vi "cs-scanning-condition-disable-example.vi"() -> ()   [LabVIEW 2017]
uses:
  raster-scan-params.ctl
  controls/PI-params.ctl
  controls/boolean_info.ctl
  <vilib>/rvi/Emulation/niFpgaGetClockAttributes.vi
  <vilib>/rvi/Emulation/niFpgaSctlEmulationGetInTimedLoop.vi
  <vilib>/rvi/Emulation/niFpgaEmulationReportErrorSimple.vi
  <vilib>/rvi/eio/common/nirviEmuTemplateMethod_errors.vi
  <vilib>/rvi/Emulation/niFpgaProcessEmulError.vi
  <vilib>/rvi/Emulation/niFpgaEmulationIsFPGAContextNoSignature.vi
  <vilib>/rvi/DataTransferAndStorage/Container/Common/niFpgaContainerGetUniqueNameForEmu.vi
  <vilib>/rvi/Memory/Memory_Emulation/niFpgaMemoryEmulationCacheClearOnFirstRun.vi
  <vilib>/rvi/Memory/Memory_Emulation/nirvimemoryEmulationManagerCache_MakeExclusive.vi
  <vilib>/rvi/Memory/Memory_Emulation/niFpgaMemoryEmulationValidateCache.vi
  <vilib>/rvi/Memory/Memory_Emulation/nirvimemoryEmulationManagerCache_InsertValue.vi
  <vilib>/Utility/error.llb/Clear Errors.vi
  <vilib>/rvi/Memory/Memory_Emulation/nirvimemoryEmulationManagerCache_ReleaseExclusive.vi
  <vilib>/rvi/Memory/Memory_Emulation/nirvimemoryEmulationManagerCache_GetValue.vi
  <vilib>/rvi/Memory/Memory_Emulation/nirvimemoryEmulationManagerCache_SetValue.vi
  <vilib>/rvi/Emulation/niFpgaCriticalErrorInLSC.vi
  <vilib>/eio/EIONode/EIONode.xnode
  <vilib>/rvi/DataTransferAndStorage/Container/XNode/niFpgaContainer.xnode
  <vilib>/rvi/DataTransferAndStorage/Register/Emulation/niFpgaRegisterEmulation.vi
  FPGA-data-logging.lvlib
  libimaging-cs.lvlib
panel:
  out "number-settled-samples-Z":i16
  in  "Z-error-threshold":sgl format="%#_13g"
  in  "Z-settled-samples\nthreshold":i16
  in  "Ki-z-absolute":sgl
  in  "z_UP 2":fxp<+/-,16,5>
  in  "z_UP":fxp<+/-,16,5>
  out "Current Case":i16
  out "boolean \nindicators":T1
  out "z-u(k)":sgl
  in  "ABORT":bool
  out "read fifo timeout":bool
  in  "u_z max":sgl
  in  "numEntities":i16
  in  "raster-scan-params":T2={"TsTicks"=1600, "Stop"=TRUE, "TOL"=0.3, "ramp-rate"=0.0, "z-u-max"=5.0, "PI-params"={"Ki"=0.001, "setpoint"=0.0}} {"z-u-max" format="%#_13g"; "TOL" format="%#_13g"}
  out "e(0) (threshhold init)":fxp<+/-,16,5>
  in  "init Z up":fxp<+/-,16,5>
  in  "trigger-0":bool
  in  "zup-N":i16
  out "number-settled-samples-y":i16
  out "number-settled-samples-x":i16
  in  "error-threshold":sgl format="%#_13g"
  in  "settled-samples\nthreshold":i16
  in  "Ki-xy":sgl=0.001 format="%#_13g"
  in  "xy-bound":sgl
  in  "initial case":i16=2
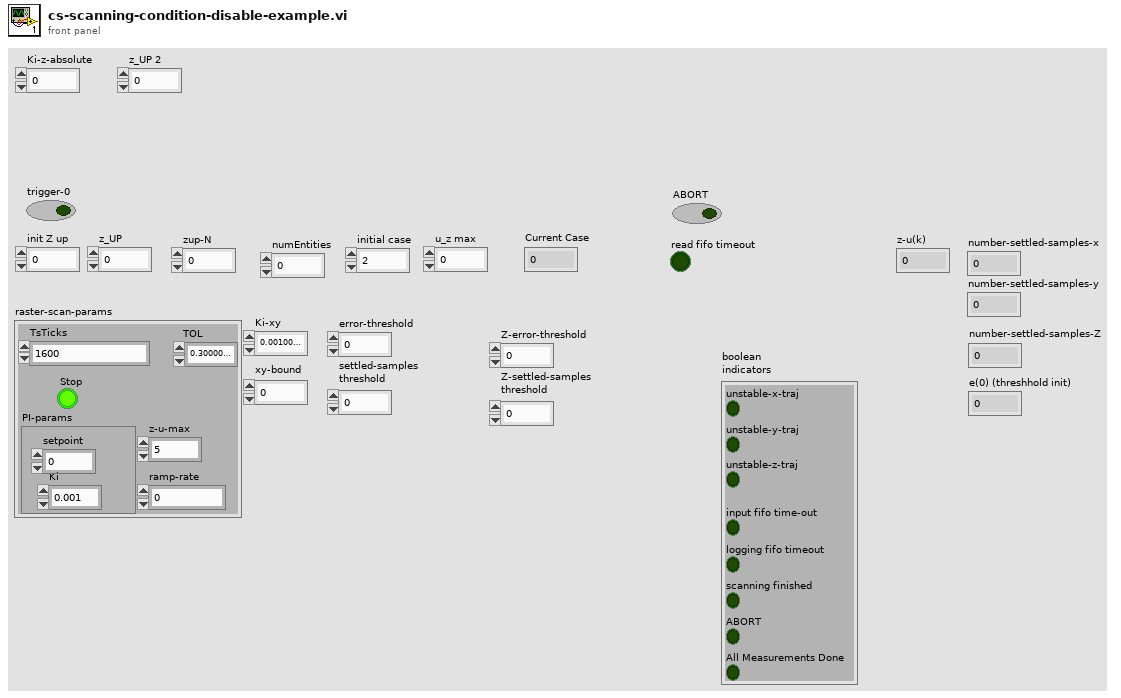
[diagram p1: front panel]
types:
  T1 = typedef "boolean_info.ctl" = cluster{"unstable-z-traj":bool, "input fifo time-out":bool, "logging fifo timeout":bool, "scanning finished":bool, "unstable-x-traj":bool, "unstable-y-traj":bool, "ABORT":bool, "All Measurements Done":bool}
  T2 = typedef "raster-scan-params.ctl" = cluster{"TsTicks":u32, "Stop":bool, "TOL":sgl, "ramp-rate":sgl, "z-u-max":sgl, "PI-params":T3}
  T3 = typedef "PI-params.ctl" = cluster{"Ki":sgl, "setpoint":sgl}
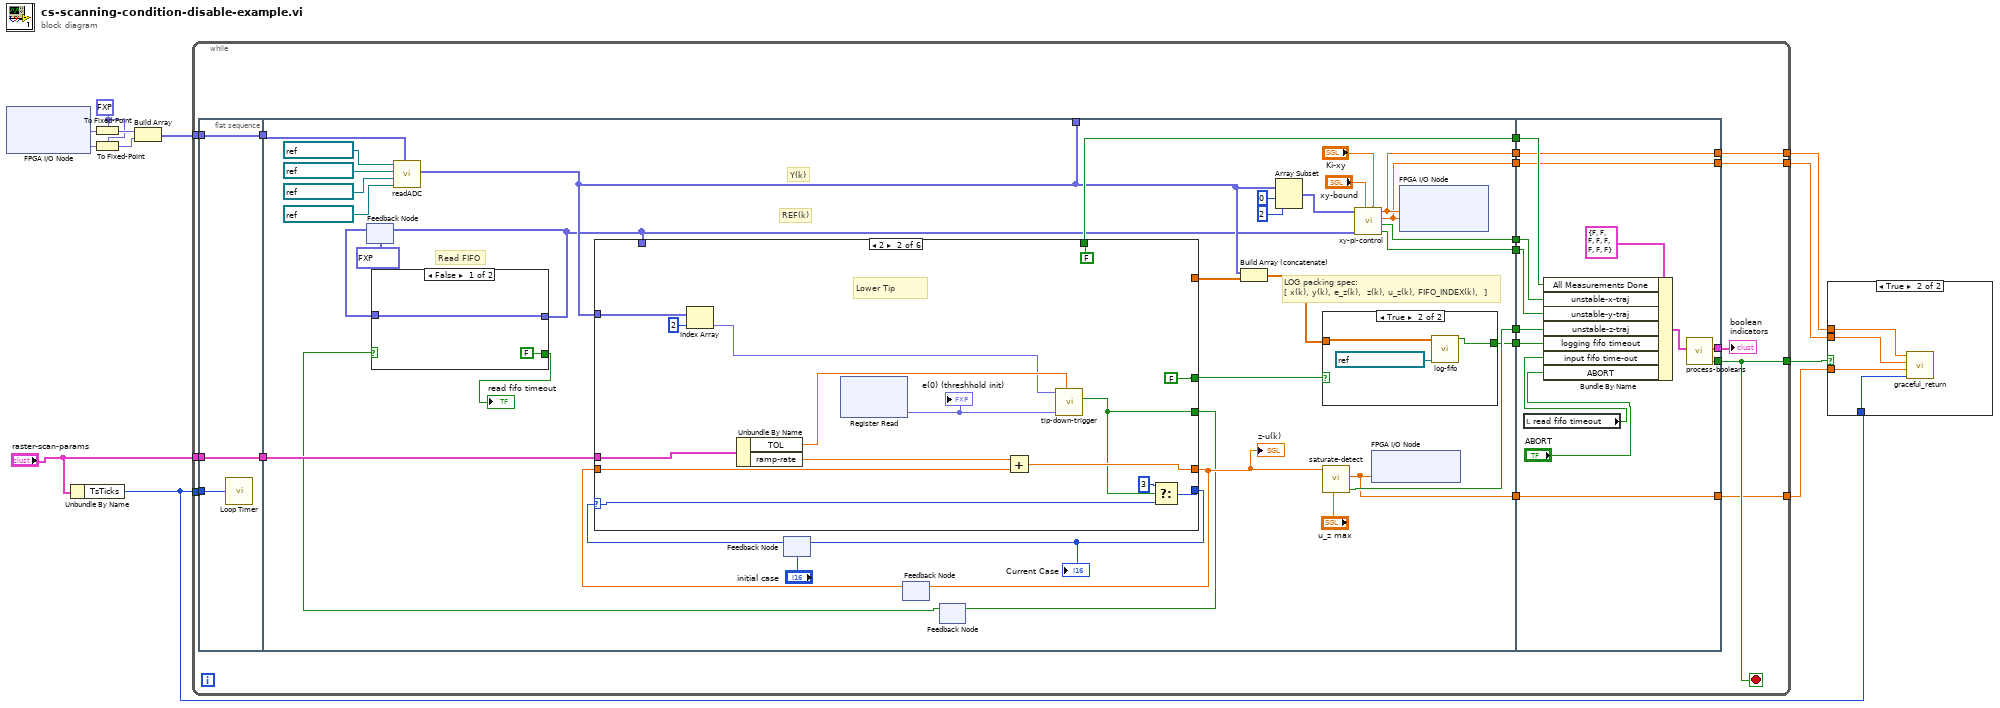
[diagram p0: block diagram]
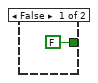
[diagram p3: hidden frame]
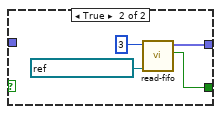
[diagram p4: hidden frame]
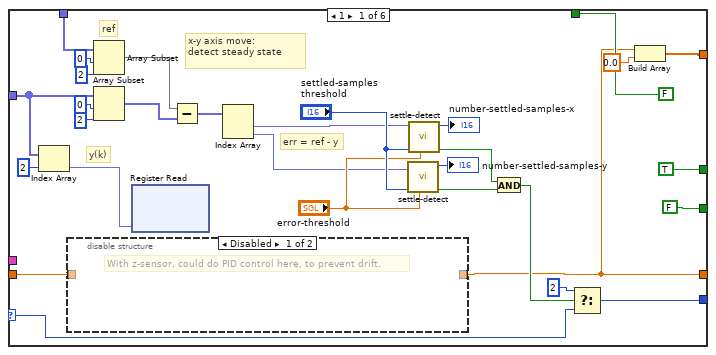
[diagram p5: hidden frame]
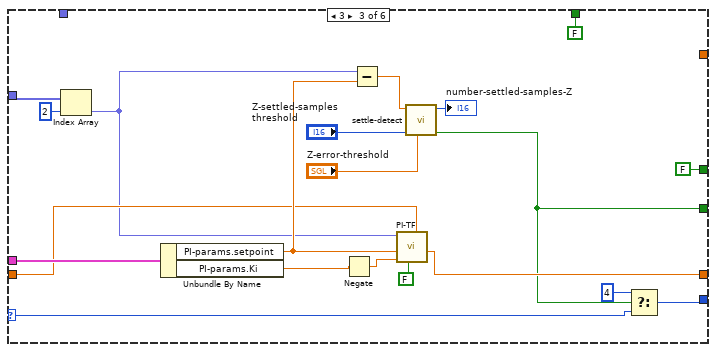
[diagram p7: hidden frame]
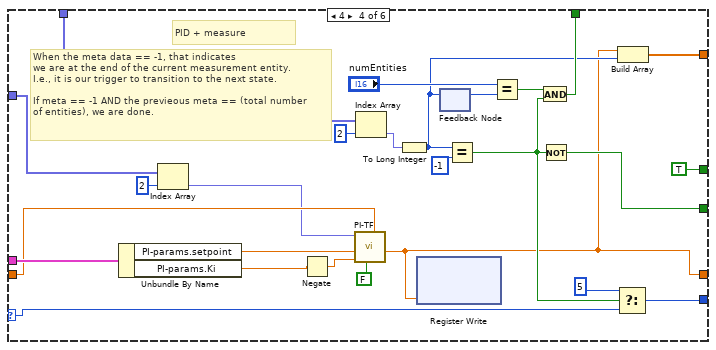
[diagram p8: hidden frame]
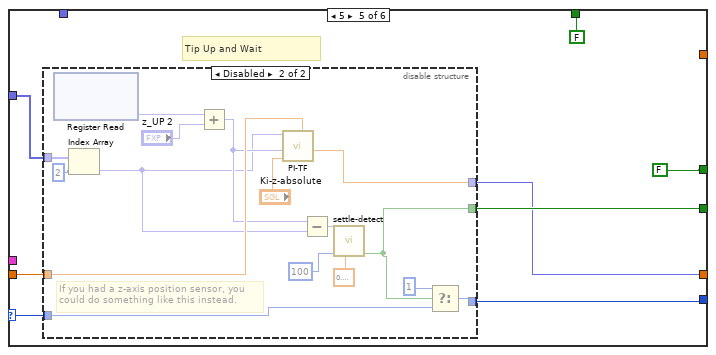
[diagram p9: hidden frame]
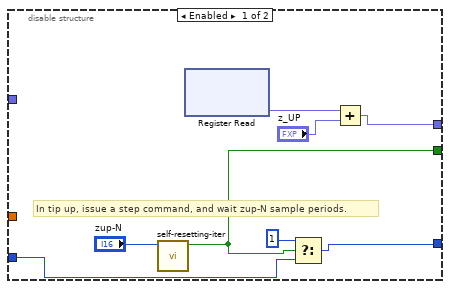
[diagram p10: hidden frame]
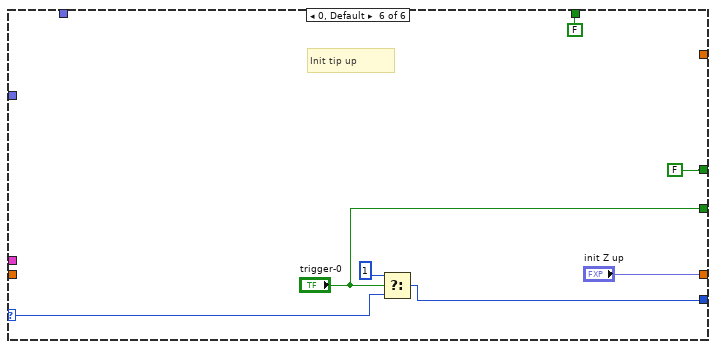
[diagram p11: hidden frame]
diagram:
  w2 = fxp<+/-,16,5> 0.0 ("fixed-point type")
  n1 = xnode "FPGA I/O Node"() -> ("Mod2/AI0"=w5:fxp<+/-,24,5>, "Mod2/AI1"=w3:fxp<+/-,24,5>)  [unwired: 2 in, 2 out]
  n2 = Unbundle By Name("raster-scan-params") -> ("TsTicks"=w1:u32)
  n3 = To Fixed-Point(fixed-point type=w2, number=w5) -> (fixed-point=w7:fxp<+/-,16,5>)
  n4 = To Fixed-Point(fixed-point type=w2, number=w3) -> (fixed-point=w4:fxp<+/-,16,5>)
  n5 = Build Array(w7, w4) -> (w6:fxp<+/-,16,5>[])
  n6 = while {
    tunnel: w6 -> [w23]
    tunnel: "raster-scan-params" -> [w22]
    tunnel: w1 -> [w21]
    tunnel: [w19] -> w11
    tunnel: [w17] -> w10
    tunnel: [w15] -> w9
    tunnel: [w13] -> w8
    stop <- w19 stop-if-true
    n7 = flat-sequence {
      tunnel: w23 -> [w33]
      tunnel: [w33] -> w30
      tunnel: w21 -> [w31]
      tunnel: w22 -> [w32]
      tunnel: [w32] -> w29
      tunnel: w30 -> [w66]
      tunnel: w29 -> [w48]
      tunnel: [w47] -> w28
      tunnel: [w46] -> w27
      tunnel: [w45] -> w26
      tunnel: [w44] -> w25
      tunnel: [w40] -> w24
      tunnel: [w39] -> _
      tunnel: [w37] -> w18
      tunnel: [w36] -> w16
      tunnel: [w35] -> w14
      tunnel: w28 -> [w223]
      tunnel: w27 -> [w222]
      tunnel: w26 -> [w221]
      tunnel: w25 -> [w218]
      tunnel: w24 -> [w215]
      tunnel: [w214] -> w19
      tunnel: [w213] -> w20
      tunnel: w18 -> [w212]
      tunnel: [w212] -> w17
      tunnel: w16 -> [w211]
      tunnel: [w211] -> w15
      tunnel: [w210] -> w13
      tunnel: w14 -> [w210]
      frame #0 {
        n8 = call "Loop Timer"("Count(Ticks)"=w31) -> ()  [unwired: 1 out]
      }
      frame #1 {
        # "REF(k)"
        # "Y(k)"
        # "LOG packing spec:\n[ x(k), y(k), e_z(k),  z(k), u_z(k), FIFO_INDEX(k),  ]"
        # "Read FIFO"
        n9 = feedback #1(fxp<+/-,16,5>[] [0.0, 0.0, 0.0] ("unpacked-data")) -> (w57:fxp<+/-,16,5>[])
        n10 = call "readADC.vi"("x(0), y(0)"=w66, "z-height"=refnum<k21> "Mod2/AI3" ("y - ADC"), "z-err- ADC"=refnum<k21> "Mod2/AI2" ("y - ADC"), "y - ADC"=refnum<k21> "Mod2/AI1", "x - ADC"=refnum<k21> "Mod2/AI0") -> ("x_y_ze_z_k"=w39:fxp<+/-,17,6>[])  [unwired: 6 in]
        n11 = feedback #2("initial case") -> (w67:i16)
        n12 = feedback #3() -> (w54:sgl)  [unwired: 1 in]
        n13 = feedback #4() -> (w41:bool)  [unwired: 1 in]
        n14 = case shown="False" w41 {
          tunnel: w57 -> [w74 _]
          tunnel: [w74 w76] -> w34
          tunnel: [FALSE ("timout?") w75] -> w43
          frame False {
          }
          frame True {
            n15 = call "read-fifo.vi"("FIFO In"=refnum<k21> "Host_to_FPGA", "numChan"=3) -> ("timout?"=w75:bool, "unpacked-data"=w76:fxp<+/-,16,5>[])  [unwired: 8 in]
          }
        }
        "read fifo timeout" <- w43
        n16 = feedback-in #1(w34) -> ()
        n17 = case shown="2" w67 {
          selector: w67 -> [w99 w121 w128 w163 w173 w207]
          tunnel: [TRUE FALSE FALSE ("trigger-0") TRUE ("trigger-0") FALSE FALSE] -> w51
          tunnel: [w100 w116 w129 w164 w172 w209] -> w56
          tunnel: w39 -> [w87 w118 w133 w146 w176 _]
          tunnel: [FALSE w112 w126 w161 w174 "trigger-0"] -> w42
          tunnel: [w92 w113 w134 w148 w171 "init Z up"] -> w52
          tunnel: w54 -> [w93 w114 w135 w158 w175 _]
          tunnel: w48 -> [_ w120 w136 w165 _ _]
          tunnel: [FALSE FALSE FALSE w151 FALSE FALSE] -> w40
          tunnel: [w94 _ _ w147 _ _] -> w50
          tunnel: w34 -> [w79 _ _ w145 _ _]
          frame 1 {
            # "err = ref - y"
            # "y(k)"
            # "ref"
            # "x-y axis move: \ndetect steady state"
            n18 = Index Array(array=w87, index=2) -> (element=w84:fxp<+/-,17,6>)
            n19 = disable-structure shown="Disabled" {
              disable-tunnel: w93 -> [_ w109]
              disable-tunnel: [_ w109] -> w92
              frame Disabled {
                # "With z-sensor, could do PID control here, to prevent drift."
              }
              frame Enabled {
              }
            }
            n20 = Array Subset(array=w79, index=0, length=2) -> (w86:fxp<+/-,16,5>[])
            n21 = Array Subset(array=w87, index=0, length=2) -> (w85:fxp<+/-,17,6>[])
            n22 = xnode ("Register Read")("Data"=w84) -> ()  [unwired: 1 in, 1 out]
            n23 = Subtract(x=w86, y=w85) -> (x-y=w82:fxp<+/-,18,7>[])
            n24 = Index Array(array=w82) -> (element #1=w81:fxp<+/-,18,7>, element #2=w80:fxp<+/-,18,7>)  [unwired: 2 in]
            n25 = call "settle-detect.vi"("error-max"="error-threshold", "settled-samples\nthreshold"="settled-samples\nthreshold", "err(k)"=w80) -> ("has-settled"=w107:bool, "number-settled-samples"=→"number-settled-samples-y":i16)  [unwired: 7 in]
            n26 = call "settle-detect.vi"("error-max"="error-threshold", "settled-samples\nthreshold"="settled-samples\nthreshold", "err(k)"=w81) -> ("has-settled"=w106:bool, "number-settled-samples"=→"number-settled-samples-x":i16)  [unwired: 7 in]
            n27 = And(x=w106, y=w107) -> (x .and. y?=w98:bool)
            n28 = Select(t=i16 2, s=w98, f=w99) -> (s? t:f=w100:i16)
            n29 = Build Array(w92, sgl 0.0 ("element")) -> (w94:sgl[])
          }
          frame 2 {
            # "Lower Tip"
            n30 = Index Array(array=w118, index=2) -> (element=w117:fxp<+/-,17,6>)
            n31 = Unbundle By Name(w120) -> ("TOL"=w123:sgl, "ramp-rate"=w122:sgl)
            n32 = xnode ("Register Read")() -> ("Data"=w124:fxp<+/-,16,5>)  [unwired: 1 in, 1 out]
            "e(0) (threshhold init)" <- w124
            n33 = Add(x=w122, y=w114) -> (x+y=w113:sgl)
            n34 = call "tip-down-trigger.vi"("TOL"=w123, "Vo"=w124, "e(k)"=w117) -> ("trigger"=w112:bool)  [unwired: 8 in]
            n35 = Select(t=i16 3, s=w112, f=w121) -> (s? t:f=w116:i16)
          }
          frame 3 {
            n36 = Index Array(array=w133, index=2) -> (element=w131:fxp<+/-,17,6>)
            n37 = Unbundle By Name(w136) -> ("PI-params.setpoint"=w138:sgl, "PI-params.Ki"=w142:sgl)
            n38 = Negate(x=w142) -> (-x=w143:sgl)
            n39 = Subtract(x=w131, y=w138) -> (x-y=w139:sgl)
            n40 = call "PI-TF.vi"("u(k-1)"=w135, "reset"=FALSE, "Ki"=w143, "setpoint"=w138, "y(k)"=w131) -> ("u(k)"=w134:sgl)  [unwired: 6 in]
            n41 = call "settle-detect.vi"("error-max"="Z-error-threshold", "settled-samples\nthreshold"="Z-settled-samples\nthreshold", "err(k)"=w139) -> ("has-settled"=w126:bool, "number-settled-samples"=→"number-settled-samples-Z":i16)  [unwired: 7 in]
            n42 = Select(t=i16 4, s=w126, f=w128) -> (s? t:f=w129:i16)
          }
          frame 4 {
            # "When the meta data == -1, that indicates\nwe are at the end of the current measurement entity.\nI.e., it is our trigger to transition to the next state.\n\nIf meta == -1 AND the previeous meta == (total number\nof entities), we are done."
            # "PID + measure"
            n43 = Unbundle By Name(w165) -> ("PI-params.setpoint"=w168:sgl, "PI-params.Ki"=w166:sgl)
            n44 = Index Array(array=w146, index=2) -> (element=w156:fxp<+/-,17,6>)
            n45 = Negate(x=w166) -> (-x=w167:sgl)
            n46 = call "PI-TF.vi"("u(k-1)"=w158, "reset"=FALSE, "Ki"=w167, "setpoint"=w168, "y(k)"=w156) -> ("u(k)"=w148:sgl)  [unwired: 6 in]
            n47 = Index Array(array=w145, index=2) -> (element=w159:fxp<+/-,16,5>)
            n48 = To Long Integer(number=w159) -> (32bit integer=w149:i32)
            n49 = xnode ("Register Write")("Data"=w148) -> ()  [unwired: 1 in, 1 out]
            n50 = feedback #5() -> (w152:i32)  [unwired: 1 in]
            n51 = feedback-in #5(w149) -> ()
            n52 = Equal?(x=w149, y=-1) -> (x = y?=w153:bool)
            n53 = Equal?(x="numEntities", y=w152) -> (x = y?=w154:bool)
            n54 = And(x=w154, y=w153) -> (x .and. y?=w151:bool)
            n55 = Not(x=w153) -> (.not. x?=w161:bool)
            n56 = Select(t=i16 5, s=w153, f=w163) -> (s? t:f=w164:i16)
            n57 = Build Array(w148, w149) -> (w147:sgl[])
          }
          frame 5 {
            # "Tip Up and Wait"
            n58 = disable-structure shown="Disabled" {
              disable-tunnel: w176 -> [_ w200]
              disable-tunnel: w175 -> [_ w197]
              disable-tunnel: [w184 w190] -> w174
              disable-tunnel: w173 -> [w183 w191]
              disable-tunnel: [w182 w192] -> w172
              disable-tunnel: [w179 w198] -> w171
              frame Enabled {
                # "In tip up, issue a step command, and wait zup-N sample periods."
                n59 = call "self-resetting-iter.vi"("N"="zup-N") -> ("Boolean"=w184:bool)  [unwired: 9 in, 1 out]
                n60 = xnode ("Register Read")() -> ("Data"=w180:fxp<+/-,16,5>)  [unwired: 1 in, 1 out]
                n61 = Select(t=i16 1, s=w184, f=w183) -> (s? t:f=w182:i16)
                n62 = Add(x=w180, y="z_UP") -> (x+y=w179:fxp<+/-,17,6>)
              }
              frame Disabled {
                # "If you had a z-axis position sensor, you\ncould do something like this instead."
                n63 = xnode ("Register Read")() -> ("Data"=w201:fxp<+/-,16,5>)  [unwired: 1 in, 1 out]
                n64 = Index Array(array=w200, index=2) -> (element=w187:fxp<+/-,17,6>)
                n65 = Add(x=w201, y="z_UP 2") -> (x+y=w188:fxp<+/-,17,6>)
                n66 = call "PI-TF.vi"("u(k-1)"=w197, "Ki"="Ki-z-absolute", "setpoint"=w188, "y(k)"=w187) -> ("u(k)"=w198:sgl)  [unwired: 7 in]
                n67 = Subtract(x=w188, y=w187) -> (x-y=w195:fxp<+/-,18,7>)
                n68 = call "settle-detect.vi"("error-max"=sgl 0.1, "settled-samples\nthreshold"=i16 100 ("settled-samples\nthreshold"), "err(k)"=w195) -> ("has-settled"=w190:bool)  [unwired: 7 in, 1 out]
                n69 = Select(t=i16 1, s=w190, f=w191) -> (s? t:f=w192:i16)
              }
            }
          }
          frame 0, Default {
            # "Init tip up"
            n70 = Select(t=i16 1, s="trigger-0", f=w207) -> (s? t:f=w209:i16)
          }
        }
        "z-u(k)" <- w52
        "Current Case" <- w56
        n71 = feedback-in #2(w56) -> ()
        n72 = feedback-in #3(w52) -> ()
        n73 = feedback-in #4(w42) -> ()
        n74 = Build Array (concatenate)(w39, w50) -> (w49:sgl[])
        n75 = Array Subset(array=w39, index=0, length=2) -> (w55:fxp<+/-,17,6>[])
        n76 = case shown="True" w51 {
          tunnel: w49 -> [_ w71]
          tunnel: [FALSE ("logging-timeout?") w70] -> w44
          frame False {
          }
          frame True {
            n77 = call "log-fifo.vi"("FIFO In"=refnum<k21> "fpga-to-host2", "input-data"=w71) -> ("logging-timeout?"=w70:bool)  [unwired: 9 in]
          }
        }
        n78 = call "saturate-detect.vi"("bound"="u_z max", "x"=w52) -> ("saturated"=w45:bool, "sat(x)"=w35:sgl)  [unwired: 8 in]
        n79 = call "xy-pi-control.vi"("Ki-xy"="Ki-xy", "xy-umax"="xy-bound", "xy-ref"=w34, "x_k-y_k"=w55) -> ("u_y saturated"=w46:bool, "u_x saturated"=w47:bool, "sat(u_y)"=w36:sgl, "sat(u_x)"=w37:sgl)  [unwired: 4 in]
        n80 = xnode "FPGA I/O Node"("Mod1/AO2"=w35) -> ()  [unwired: 1 in, 1 out]
        n81 = xnode "FPGA I/O Node"("Mod1/AO0"=w37, "Mod1/AO1"=w36) -> ()  [unwired: 2 in, 2 out]
      }
      frame #2 {
        n82 = local read "read fifo timeout"() -> (w217:bool)
        n83 = Bundle By Name(cluster=T1 {"unstable-z-traj"=FALSE, "input fifo time-out"=FALSE, "logging fifo timeout"=FALSE, "scanning finished"=FALSE, "unstable-x-traj"=FALSE, "unstable-y-traj"=FALSE, "ABORT"=FALSE, "All Measurements Done"=FALSE} ("boolean errors"), "All Measurements Done"=w215, "unstable-x-traj"=w223, "unstable-y-traj"=w222, "unstable-z-traj"=w221, "logging fifo timeout"=w218, "input fifo time-out"=w217, "ABORT"="ABORT") -> (w219:T1)
        n84 = call "process-booleans.vi"("boolean indicators 2"=w219) -> ("scaning finished"=w214:bool, "boolean indicators"=w213:T1)  [unwired: 9 in]
      }
    }
    "boolean \nindicators" <- w20
  }
  n85 = case shown="True" w11 {
    tunnel: w1 -> [_ w227]
    tunnel: w10 -> [_ w226]
    tunnel: w9 -> [_ w225]
    tunnel: w8 -> [_ w224]
    frame False {
    }
    frame True {
      n86 = call "graceful_return.vi"("TsTicks"=w227, "uz(0)"=w224, "uy(0)"=w225, "ux(0)"=w226) -> ()  [unwired: 8 in]
    }
  }
